vi "theta2zpk.vi"(7 "Sampling Time (s)":dbl=4e-05 format="%#_13g", 11 "theta in":dbl[](array[numeric])) -> (3 "Model Out":T1 {"zero-pole-gain(s)"."delay" format="%.4f"; "zero-pole-gain(s)"."Poles" format="%#.8g"; "zero-pole-gain(s)"."Zeros" format="%#.8g"; "zero-pole-gain(s)"."Gain" format="%#.8g"; "properties"."Sampling Time" format="%#.6p"; "properties"."Output Delays" format="%.4f"; "properties"."Input Delays" format="%.4f"})   [LabVIEW 2017]
uses:
  <vilib>/addons/Control Design/_Model Construction/Model Typedefs.llb/CD Zero-Pole-Gain Model (MIMO).ctl
  <vilib>/addons/Control Design/_Model Construction/Model Typedefs.llb/CD General Elements.ctl
  <vilib>/addons/Control Design/_Model Construction/Model Typedefs.llb/CD Zero-Pole-Gain Model (SISO).ctl
  <vilib>/addons/Control Design/_Model Construction/Model Creation.llb/Model Creation SubVI/cd_Create Zero-Pole-Gain Model.vi
  <vilib>/addons/Control Design/_Model Construction/Model Creation.llb/Model Creation SubVI/cd_Create Transfer Function Model.vi
  <vilib>/addons/Control Design/_Model Conversions/Model Type.llb/Model Conversion SubVI/cd_Convert Transfer Function to Zero-Pole-Gain Model.vi
  <vilib>/addons/Control Design/_Model Interconnection/Model Interconnection.llb/Model Interconnection SubVI/cd_Matrix Multiply Models (ZPK and ZPK).vi
  <vilib>/addons/Control Design/_Model Construction/NI_LinSys_Model Creation.lvlib
  <vilib>/addons/Control Design/_Model Conversions/NI_CD_Model Type.lvlib
  <vilib>/addons/Control Design/_Model Interconnection/NI_CD_Model Interconnection.lvlib
  <vilib>/addons/Control Design/_Model Construction/NI_LinSys_Model Typedefs.lvlib
panel:
  out "error out":errorcluster
  in  "error in (no error)":errorcluster
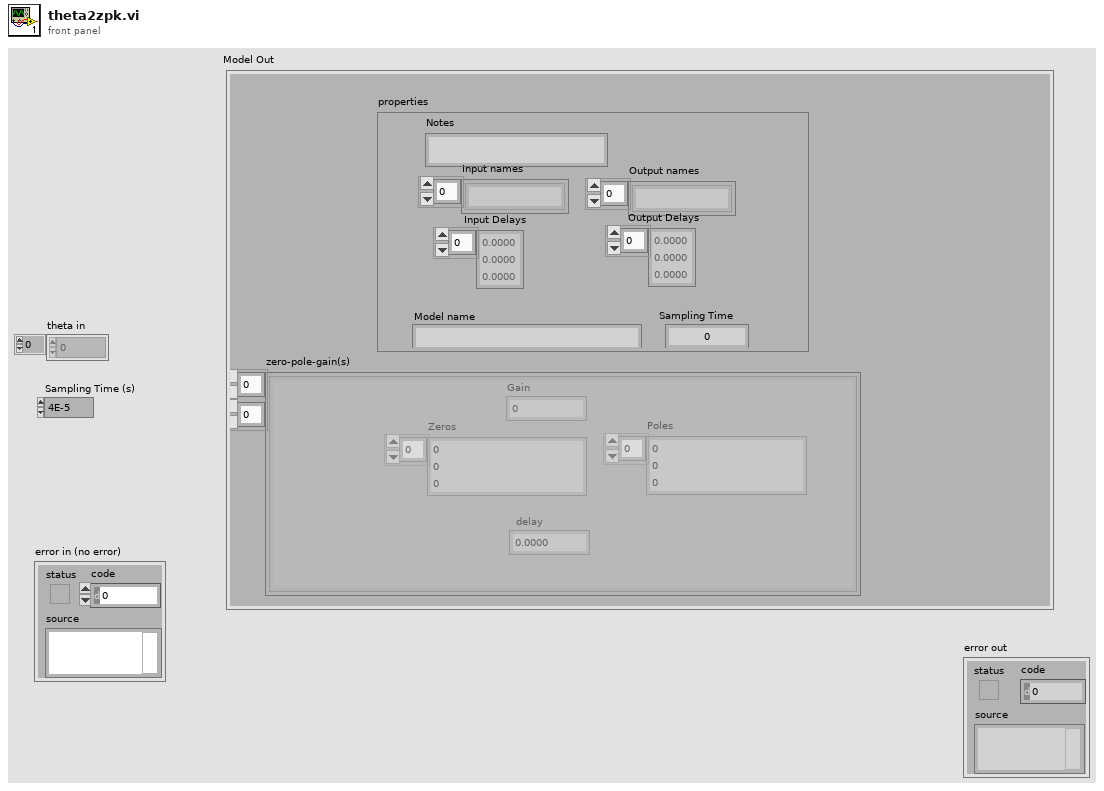
[diagram p1: front panel]
types:
  T1 = typedef "NI_LinSys_Model Typedefs.lvlib/CD Zero-Pole-Gain Model (MIMO).ctl" = cluster{"properties":T2, "zero-pole-gain(s)":T3[][]}
  T2 = typedef "NI_LinSys_Model Typedefs.lvlib/CD General Elements.ctl" = cluster{"Model name":string, "Input names":string[], "Output names":string[], "Input Delays":dbl[], "Output Delays":dbl[], "Sampling Time":dbl, "Notes":string}
  T3 = typedef "NI_LinSys_Model Typedefs.lvlib/CD Zero-Pole-Gain Model (SISO).ctl" = cluster{"Gain":dbl, "Zeros":cdb[], "Poles":cdb[], "delay":dbl}
  T4 = typedef "NI_LinSys_Model Typedefs.lvlib/CD Transfer Function Model (MIMO).ctl" = cluster{"properties":T2, "transfer function(s)":T5[][]}
  T5 = typedef "NI_LinSys_Model Typedefs.lvlib/CD Transfer Function Model (SISO).ctl" = cluster{"Numerator":dbl[], "Denominator":dbl[], "delay":dbl}
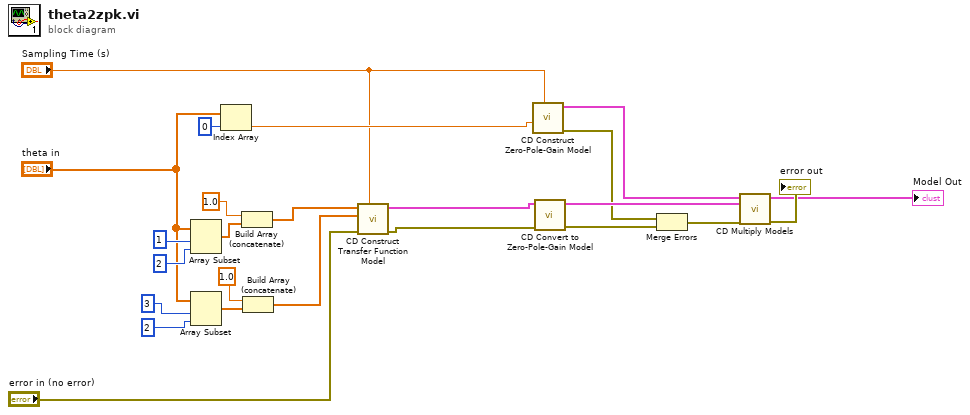
[diagram p0: block diagram]
diagram:
  n1 = Array Subset(array="theta in", index=1, length=2 ("index")) -> (w6:dbl[])
  n2 = Array Subset(array="theta in", index=3, length=2 ("index")) -> (w4:dbl[])
  n3 = Index Array(array="theta in", index=0) -> (element=w14:dbl)
  n4 = Build Array (concatenate)(1.0, w6) -> (w1:dbl[])
  n5 = Build Array (concatenate)(1.0, w4) -> (w2:dbl[])
  n6 = call-poly <vilib>:"CD Construct Transfer Function Model.vi"("Sampling Time (s)"="Sampling Time (s)", "error in (no error)"="error in (no error)", "Denominator"=w2, "Numerator"=w1) -> ("error out"=w17:errorcluster, "Transfer Function Model"=w24:T4)  [unwired: 6 in]
  n7 = call-poly <vilib>:"CD Construct Zero-Pole-Gain Model.vi"("Sampling Time (s)"="Sampling Time (s)", "Gain"=w14) -> ("error out"=w10:errorcluster, "Zero-Pole-Gain Model"=w13:T1)  [unwired: 8 in]
  n8 = call-poly <vilib>:"CD Convert to Zero-Pole-Gain Model.vi"("error in (no error)"=w17, "Transfer Function Model"=w24) -> ("error out"=w11:errorcluster, "Zero-Pole-Gain Model"=w15:T1)  [unwired: 8 in]
  n9 = Merge Errors(w10, w11) -> (w12:errorcluster)
  n10 = call-poly <vilib>:"CD Multiply Models.vi"("error in (no error)"=w12, "Model 2"=w15, "Model 1"=w13) -> ("error out"=→"error out":errorcluster, "Model Out"=→"Model Out":T1)  [unwired: 7 in]
